vi "connect.vi"(10 "T button?":bool, 11 "Delacor_lib_QMH_Message Queue in":refnum<class "Delacor_lib_QMH_Message Queue.lvclass">) -> (0 "error out":errorcluster)   [LabVIEW 2020, in "Serial Device.lvlib"]
uses:
  Serial Device.lvlib
  <vilib>/Delacor/Delacor QMH/Libraries/Message Queue_class/Delacor_lib_QMH_Message Queue.lvclass
  <vilib>/Delacor/Delacor QMH/Libraries/Message Queue_class/Delacor_lib_QMH_Message Queue.lvclass/Delacor_lib_QMH_Message Queue.ctl
  <vilib>/Delacor/Delacor QMH/Libraries/Message Queue_class/Delacor_lib_QMH_Enqueue Message (Single).vi
panel:
  in  "Exit":bool
  in  "VISA resource name":refnum<visa-resource-name>
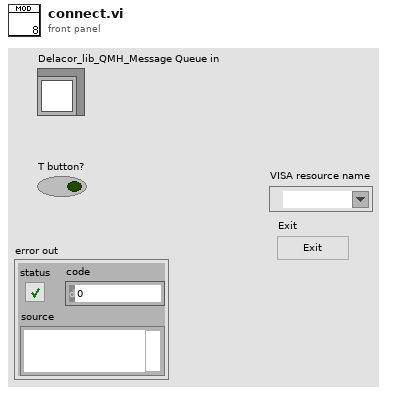
[diagram p1: front panel]
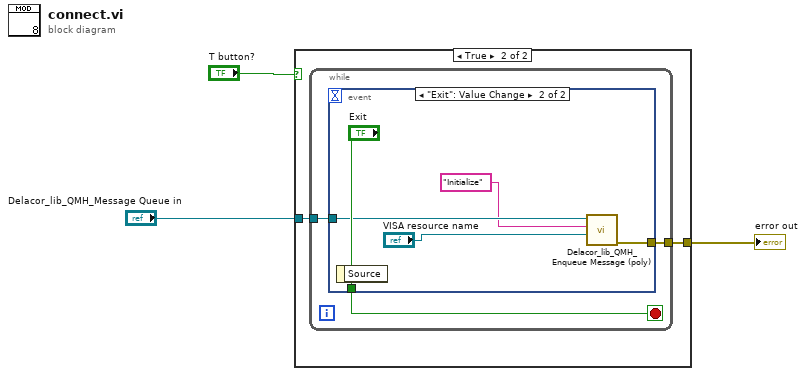
[diagram p0: block diagram]
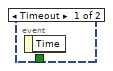
[diagram p3: hidden frame]
diagram:
  n1 = case shown="True" "T button?" {
    tunnel: "Delacor_lib_QMH_Message Queue in" -> [_ w5]
    tunnel: [_ w4] -> w1
    frame False {
    }
    frame True {
      n2 = while {
        tunnel: w5 -> [w7]
        tunnel: [w6] -> w4
        stop <- w8 stop-if-true
        n3 = event shown="[1] \"Exit\": Value Change" {
          selector: _ -> [_ _]
          dyn-events: _ -> [_ _]
          timeout: _ -> [_ _]
          tunnel: [_ "Exit"] -> w8
          tunnel: w7 -> [_ w12]
          tunnel: [_ w9] -> w6
          event Timeout {
            n4 = event-data() -> ()  [unwired: 1 in, 1 out]
          }
          event "Exit": Value Change {
            n5 = event-data() -> ()  [unwired: 1 in, 1 out]
            n6 = call-poly <vilib>:"Delacor_lib_QMH_Enqueue Message (poly).vi"("Message Data"="VISA resource name", "Message"="Initialize", "Message Queue in"=w12) -> ("error out"=w9:errorcluster)  [unwired: 7 in, 1 out]
          }
        }
      }
    }
  }
  "error out" <- w1
